vi "Rename Project.vi"(8 "error in (no error)":errorcluster, 11 "ProjectItem in":refnum<class "ProjectItem.lvclass">) -> (0 "error out":errorcluster, 3 "ProjectItem out":refnum<class "ProjectItem.lvclass">)   [LabVIEW 2019, in "ProjectItem.lvclass"]
uses:
  ProjectItem.lvclass
  ProjectItem.lvclass/ProjectItem.ctl
panel:
  out "Project Name":string
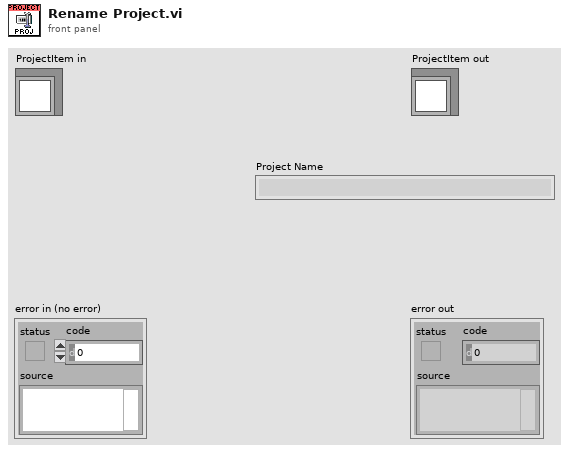
[diagram p1: front panel]
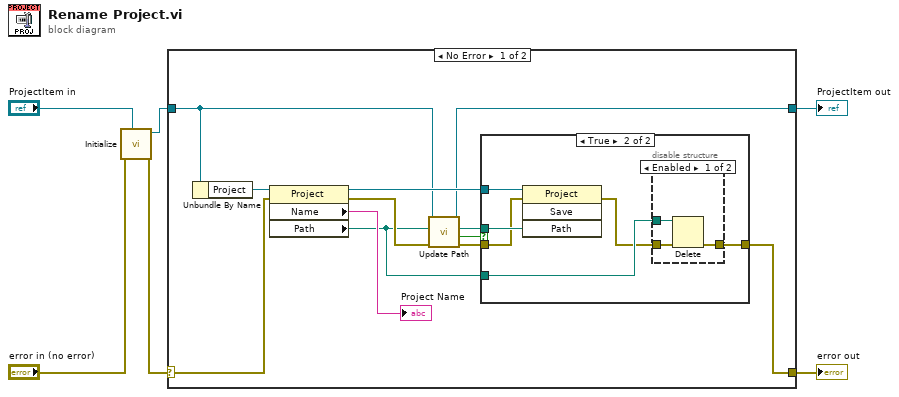
[diagram p0: block diagram]
diagram:
  n1 = call "Initialize.vi"("ProjectItem"="ProjectItem in", "error in (no error)"="error in (no error)") -> ("error out"=w1:errorcluster, "ProjectItem out"=w3:refnum<class "ProjectItem.lvclass">)  [unwired: 8 in]
  n2 = case shown="No Error" w1 {
    selector: w1 -> [w15 w31]
    tunnel: [w7 w31] -> w6
    tunnel: [w14 w30] -> w5
    tunnel: w3 -> [w12 w30]
    frame No Error {
      n3 = Unbundle By Name(w12) -> ("Project"=w16:refnum<vi>)
      n4 = property class="Project"(reference=w16, error in=w15) -> (reference out=w17:refnum<vi>, error out=w11:errorcluster, "Name"=→"Project Name":string, "Path"=w8:path)
      n5 = call "Update Path.vi"("error in (no error)"=w11, "Path in"=w8, "Rename in"=w12) -> ("error out"=w10:errorcluster, "New Path?"=w9:bool, "Path out"=w18:path, "Rename out"=w14:refnum<class "ProjectItem.lvclass">)  [unwired: 5 in]
      n6 = case shown="True" w9 {
        tunnel: w18 -> [_ w25]
        tunnel: w17 -> [_ w24]
        tunnel: [w19 w22] -> w7
        tunnel: w10 -> [w19 w23]
        tunnel: w8 -> [_ w21]
        frame False {
        }
        frame True {
          n7 = invoke class="Project" method="Save"(reference=w24, error in=w23, "Path"=w25) -> (error out=w20:errorcluster)  [unwired: 1 in, 3 out]
          n8 = disable-structure shown="Enabled" {
            disable-tunnel: w21 -> [w28 _]
            disable-tunnel: w20 -> [w27 w29]
            disable-tunnel: [w26 w29] -> w22
            frame Enabled {
              n9 = Delete(path (use dialog)=w28, error in=w27) -> (error out=w26:errorcluster)  [unwired: 3 in, 2 out]
            }
            frame Disabled {
            }
          }
        }
      }
    }
    frame Error {
    }
  }
  "error out" <- w6
  "ProjectItem out" <- w5
